vi "GetClassProperties.vi"(0 "reference in":refnum<class "ClassWriterGOOP300.lvclass">, 1 "LvClassItem":refnum<vi>, 2 "TreeControl":refnum<vi>, 5 "error in (no error)":errorcluster) -> (14 "reference out":refnum<class "ClassWriterGOOP300.lvclass">, 19 "error out":errorcluster)   [LabVIEW 2014, in "ClassWriterGOOP300.lvclass"]
uses:
  <resource>/Framework/Providers/Open_GDS/ClassProviders/Provider_EndevoGOOP300/ClassWriterGOOP300_class/ClassWriterGOOP300.lvclass
panel:
  out "ClassClasses":string[](array[string])
  out "ObjectClasses":string[](array[string])
  out "ClassAttributes":string[][](array[string])
  out "ObjectAttributes":string[][](array[string])
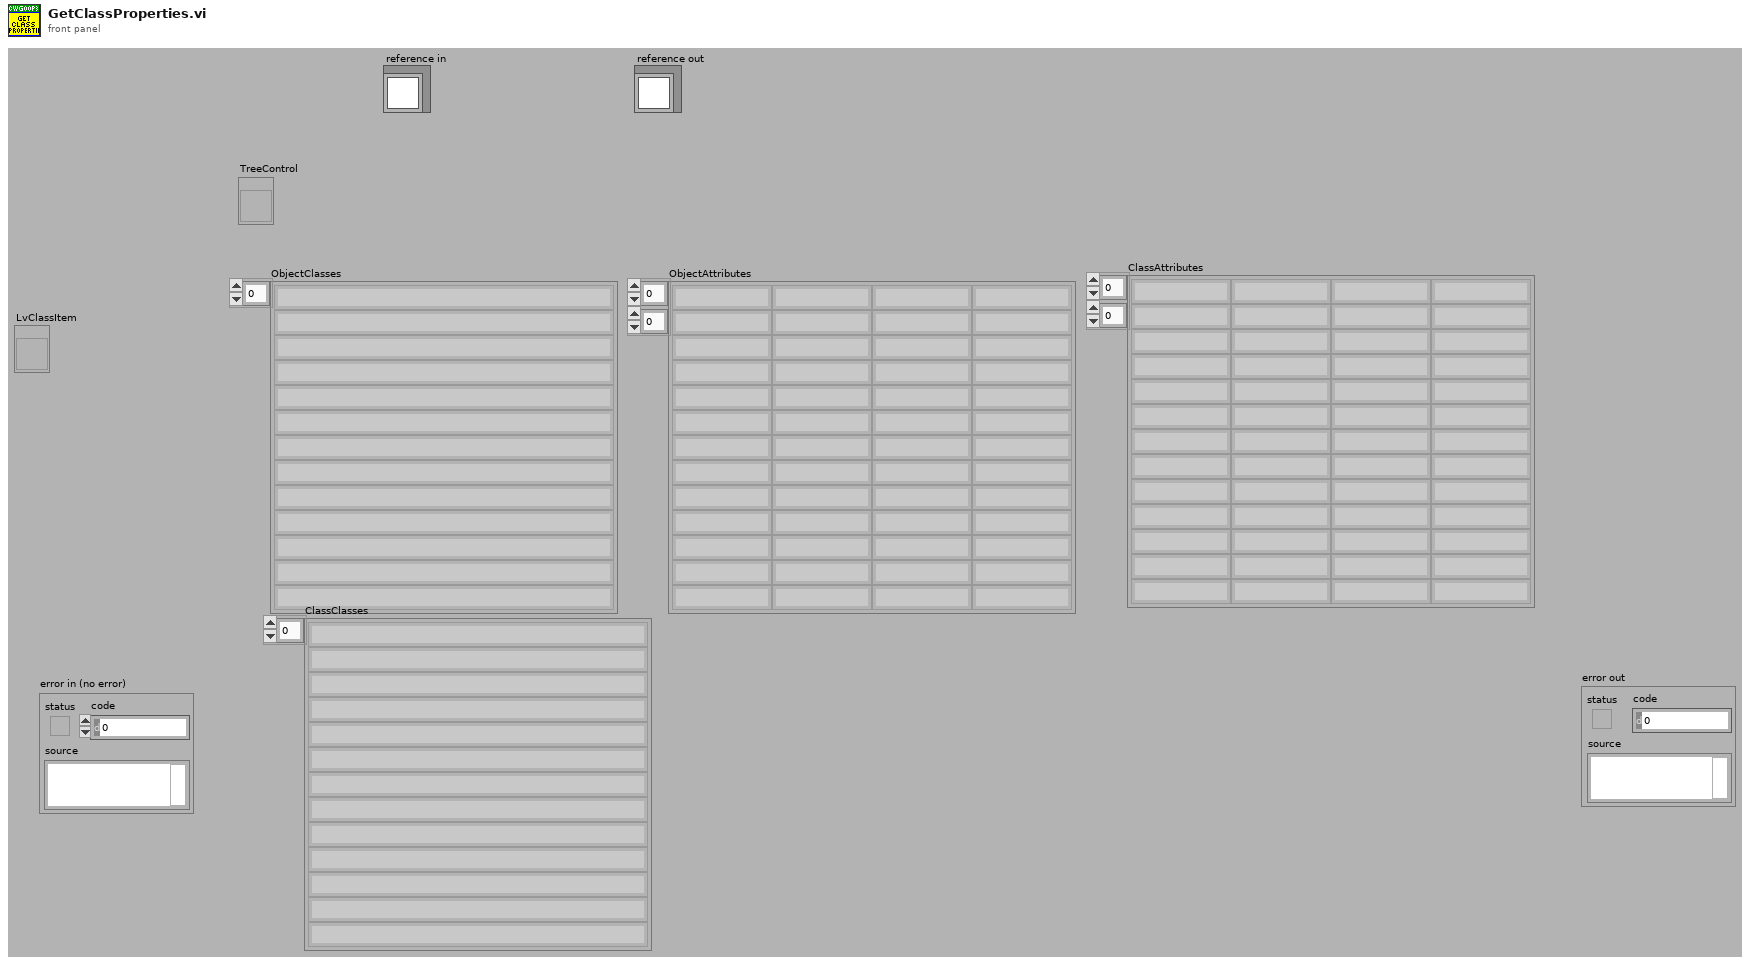
[diagram p1: front panel]
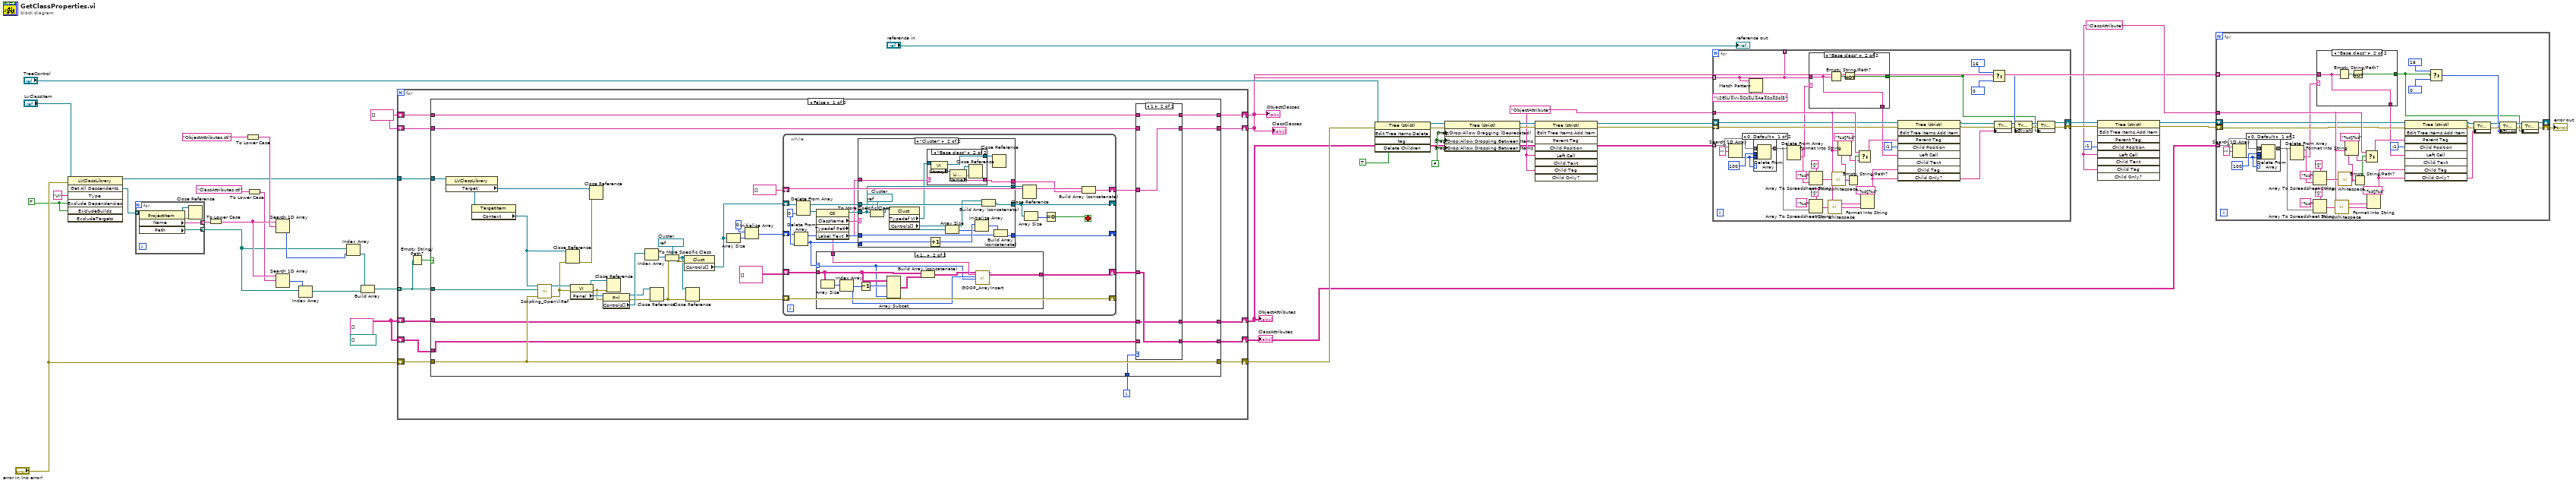
[diagram p0: block diagram]
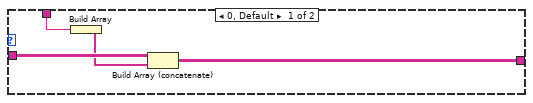
[diagram p7: hidden frame]
diagram:
  w2 = TRUE ("ExcludeDependencies")
  w10 = "ClassAttribute" ("Left Cell String(Main name)")
  w19 = FALSE ("Drag/Drop:Allow Dragging (Deprecated)")
  w13 = "ObjectAttribute" ("Left Cell String(Main name)")
  w25 = string[] []
  (unwired) path[] []
  w42 = string[][] []
  n1 = invoke class="LVClassLibrary" method="Get All Descendents"(reference="LvClassItem", error in="error in (no error)", "Type"="VI", "Exclude Dependencies"=w2, "ExcludeBuilds"=w2) -> (reference out=w1:refnum<vi>, "All Descendents"=w40:refnum<vi>[])  [unwired: 2 in, 5 out]
  n2 = for {
    tunnel: w40 -> [w48] mode=indexing
    tunnel: [w47] -> w39 mode=indexing
    tunnel: [w46] -> w33 mode=indexing
    n3 = property class="ProjectItem"(reference=w48) -> (reference out=w45:refnum<vi>, error out=w44:errorcluster, "Name"=w47:string, "Path"=w46:path)  [unwired: 1 in]
    n4 = Close Reference(reference=w45, error in (no error)=w44) -> ()  [unwired: 1 out]
  }
  n5 = To Lower Case(string=w39) -> (all lower case string=w37:string[])
  n6 = To Lower Case(string="ObjectAttributes.ctl") -> (all lower case string=w38:string)
  n7 = To Lower Case(string="ClassAttributes.ctl") -> (all lower case string=w36:string)
  n8 = Search 1D Array(1D array=w37, element=w38) -> (index of element=w35:i32)  [unwired: 1 in]
  n9 = Search 1D Array(1D array=w37, element=w36) -> (index of element=w34:i32)  [unwired: 1 in]
  n10 = Index Array(array=w33, index=w34) -> (element=w27:path)
  n11 = Index Array(array=w33, index=w35) -> (element=w28:path)
  n12 = Build Array(w28, w27) -> (w32:path[])
  n13 = for {
    shift-right: [w62] -> w7
    shift-left: "error in (no error)" -> [w61]
    shift-right: [w59] -> w6
    shift-left: w42 -> [w60]
    shift-right: [w57] -> w5
    shift-left: w42 -> [w58]
    tunnel: w32 -> [w56] mode=indexing
    shift-right: [w53] -> w4
    shift-left: w25 -> [w50]
    shift-right: [w52] -> w3
    shift-left: w25 -> [w51]
    tunnel: w1 -> [w49]
    i -> [w54]
    n14 = Empty String/Path?(string/path=w56) -> (empty?=w55:bool)
    n15 = case shown="False" w55 {
      tunnel: [w97 w171] -> w62
      tunnel: w61 -> [w97 w171]
      tunnel: w60 -> [w81 w172]
      tunnel: [w84 w172] -> w59
      tunnel: w58 -> [w83 w170]
      tunnel: [w82 w170] -> w57
      tunnel: w56 -> [w99 _]
      tunnel: w54 -> [w86 _]
      tunnel: [w72 w169] -> w53
      tunnel: [w70 w168] -> w52
      tunnel: w51 -> [w69 w168]
      tunnel: w50 -> [w68 w169]
      tunnel: w49 -> [w67 _]
      frame False {
        w90 = refnum<vi> refnum  # Cluster
        n16 = property class="LVClassLibrary"(reference=w67) -> ("Target"=w64:refnum<vi>)  [unwired: 1 in, 2 out]
        n17 = property class="TargetItem"(reference=w64) -> ("Context"=w66:refnum<vi>)  [unwired: 1 in, 2 out]
        n18 = call <resource>:"Scripting_OpenViRef.vi"("error in"=w97, "ViPath/ViName/Viref"=w99, "AppRef"=w66) -> ("error out"=w65:errorcluster, "vi reference"=w98:refnum<vi>)  [unwired: 6 in, 1 out]
        n19 = Close Reference(reference=w66, error in (no error)=w65) -> (error out=w63:errorcluster)
        n20 = property class="VI"(reference=w98, error in=w65) -> (reference out=w79:refnum<vi>, error out=w80:errorcluster, "Panel"=w96:refnum<vi>)
        n21 = Close Reference(reference=w64, error in (no error)=w63) -> ()  [unwired: 1 out]
        n22 = property class="Pnl"(reference=w96, error in=w80) -> (reference out=w74:refnum<vi>, error out=w76:errorcluster, "Controls[]"=w91:refnum<vi>[])
        n23 = Close Reference(reference=w79, error in (no error)=w80) -> ()  [unwired: 1 out]
        n24 = Index Array(array=w91) -> (element=w89:refnum<vi>)  [unwired: 1 in]
        n25 = Close Reference(reference=w74, error in (no error)=w76) -> (error out=w75:errorcluster)
        n26 = To More Specific Class(target class=w90, reference=w89, error in=w75) -> (specific class reference=w78:refnum<vi>, error out=w88:errorcluster)
        n27 = property class="Clust"(reference=w78, error in=w88) -> ("Controls[]"=w87:refnum<vi>[])  [unwired: 2 out]
        n28 = Close Reference(reference=w78, error in (no error)=w75) -> (error out=w77:errorcluster)
        n29 = Array Size(array=w87) -> (size(s)=w94:i32)
        n30 = Initialize Array(0 ("index"), w94) -> (w92:i32[])
        n31 = while {
          shift-right: [w126] -> _
          shift-left: w87 -> [w128]
          shift-right: [w113] -> _
          shift-left: w77 -> [w113]
          shift-right: [w121] -> w85
          shift-left: string[][] [] -> [w122]
          shift-right: [w115] -> _
          shift-left: w92 -> [w117]
          shift-right: [w110] -> w71
          shift-left: string[] [] -> [w111]
          stop <- w124 stop-if-true
          w118 = 0 ("index")
          n32 = Delete From Array(array=w117, index=w118) -> (deleted portion=w114:i32, array with subset deleted=w116:i32[])  [unwired: 1 in]
          n33 = Delete From Array(array=w128, index=w118) -> (deleted portion=w123:refnum<vi>, array with subset deleted=w127:refnum<vi>[])  [unwired: 1 in]
          n34 = property class="Ctl" props=["ClassName", "Typedef Path", "Label", "Text"](reference=w123) -> (reference out=w119:refnum<vi>, "ClassName"=w120:string, "Label.Text"=w108:string)  [unwired: 1 in, 2 out]
          n35 = case shown="1.." w114 {
            selector: w114 -> [_ w133]
            tunnel: w122 -> [w132 w137]
            tunnel: [w131 w140] -> w121
            tunnel: w108 -> [w130 w139]
            frame 0, Default {
              n36 = Build Array(w130) -> (w129:string[])
              n37 = Build Array (concatenate)(w132, w129) -> (w131:string[][])
            }
            frame 1.. {
              n38 = Array Size(array=w137) -> (size(s)=w141:i32[])
              n39 = Index Array(array=w141) -> (element=w135:i32)  [unwired: 1 in]
              n40 = Decrement(x=w135) -> (x-1=w134:i32)
              n41 = Array Subset(array=w137, index (row)=w134, length (col)=w133) -> (w136:string[][])  [unwired: 2 in]
              n42 = Build Array (concatenate)(w137, w136) -> (w138:string[][])
              n43 = call <resource>:"GOOP_ArrayInsert.vi"("ArrayIn"=w138, "Text"=w139, "Row"=w135, "Column"=w133) -> ("ArrayOut"=w140:string[][])  [unwired: 15 in]
            }
          }
          n44 = case shown="\"Cluster\"" w120 {
            tunnel: [w144 w158] -> w126
            tunnel: w127 -> [w144 w157]
            tunnel: w119 -> [w142 w149]
            tunnel: w116 -> [w143 w151]
            tunnel: [w143 w152] -> w115
            tunnel: w114 -> [_ w155]
            tunnel: [w142 w149] -> w112
            tunnel: [_ w147] -> w109
            tunnel: w108 -> [_ w145]
            frame Default {
            }
            frame "Cluster" {
              w160 = refnum<vi> refnum  # Cluster
              n45 = To More Specific Class(target class=w160, reference=w149) -> (specific class reference=w159:refnum<vi>)  [unwired: 1 in, 1 out]
              n46 = property class="Clust"(reference=w159) -> ("Typedef VI"=w148:refnum<vi>, "Controls[]"=w156:refnum<vi>[])  [unwired: 1 in, 2 out]
              n47 = case shown="\"Base class\"" w145 {
                tunnel: w148 -> [w161 w167]
                tunnel: [_ w165] -> w147
                tunnel: [w161 w162] -> w146
                frame "False", Default {
                }
                frame "Base class" {
                  n48 = property class="VI"(reference=w167) -> (reference out=w162:refnum<vi>, "Library"=w166:refnum<vi>)  [unwired: 1 in, 1 out]
                  n49 = property class="Library"(reference=w166) -> (reference out=w164:refnum<vi>, error out=w163:errorcluster, "Name"=w165:string)  [unwired: 1 in]
                  n50 = Close Reference(reference=w164, error in (no error)=w163) -> ()  [unwired: 1 out]
                }
              }
              n51 = Increment(x=w155) -> (x+1=w154:i32)
              n52 = Array Size(array=w156) -> (size(s)=w153:i32)
              n53 = Initialize Array(w154, w153) -> (w150:i32[])
              n54 = Build Array (concatenate)(w156, w157) -> (w158:refnum<vi>[])
              n55 = Close Reference(reference=w146) -> ()  [unwired: 1 in, 1 out]
              n56 = Build Array (concatenate)(w150, w151) -> (w152:i32[])
            }
          }
          n57 = Close Reference(reference=w112) -> ()  [unwired: 1 in, 1 out]
          n58 = Array Size(array=w126) -> (size(s)=w125:i32)
          n59 = Equal To 0?(x=w125) -> (x = 0?=w124:bool)
          n60 = Build Array (concatenate)(w111, w109) -> (w110:string[])
        }
        n61 = case shown="1" w86 {
          tunnel: [w103 w106] -> w84
          tunnel: w85 -> [w103 w107]
          tunnel: w83 -> [w102 _]
          tunnel: [w102 w107] -> w82
          tunnel: w81 -> [_ w106]
          tunnel: [w101 w105] -> w72
          tunnel: w71 -> [w101 w104]
          tunnel: [w100 w104] -> w70
          tunnel: w69 -> [w100 _]
          tunnel: w68 -> [_ w105]
          frame 0, Default {
          }
          frame 1 {
          }
        }
      }
      frame True {
      }
    }
  }
  "ObjectAttributes" <- w6
  "ClassAttributes" <- w5
  "ObjectClasses" <- w4
  "ClassClasses" <- w3
  n62 = invoke on="Invoke Node" class="Tree (strict)" method="Edit Tree Items.Delete"(reference="TreeControl", error in=w7, "Delete Children"=TRUE) -> (reference out=w23:refnum<vi>, error out=w22:errorcluster)  [unwired: 2 in, 3 out]
  n63 = property class="Tree (strict)"(reference=w23, error in=w22, "Drag/Drop:Allow Dragging (Deprecated)"=w19, "Drag/Drop:Allow Dropping Between Items"=w19, "Drag/Drop:Allow Dropping Between Items"=w19) -> (reference out=w21:refnum<vi>, error out=w20:errorcluster)
  n64 = invoke on="Invoke Node" class="Tree (strict)" method="Edit Tree Items.Add Item"(reference=w21, error in=w20, "Left Cell"=w13, "Child Tag"=w13) -> (reference out=w12:refnum<vi>, error out=w11:errorcluster)  [unwired: 5 in, 7 out]
  n65 = for {
    shift-right: [w175] -> w17
    shift-left: w11 -> [w192]
    shift-right: [w174] -> w18
    shift-left: w12 -> [w191]
    tunnel: w6 -> [w211] mode=indexing
    tunnel: w13 -> [w194]
    tunnel: w4 -> [w181] mode=indexing
    tunnel: [w181] -> _ mode=indexing
    n66 = Search 1D Array(1D array=w211, element="") -> (index of element=w200:i32)  [unwired: 1 in]
    n67 = Match Pattern(string=w181, regular expression="\\2E[Ll][Vv][Cc][Ll][Aa][Ss][Ss]$") -> ()  [unwired: 1 in, 4 out]
    n68 = case shown="0, Default" w200 {
      tunnel: w200 -> [w220 _]
      tunnel: w211 -> [w219 w221]
      tunnel: 100 ("length") -> [w218 _]
      tunnel: [w217 w221] -> w201
      frame 0, Default {
        n69 = Delete From Array(array=w219, length=w218, index=w220) -> (array with subset deleted=w217:string[])  [unwired: 1 out]
      }
      frame -1 {
      }
    }
    n70 = Delete From Array(array=w201) -> (deleted portion=w189:string, array with subset deleted=w209:string[])  [unwired: 2 in]
    n71 = case shown="\"Base class\"" w189 {
      selector: w189 -> [w213 _]
      tunnel: [w213 w214] -> w188
      tunnel: w181 -> [_ w214]
      tunnel: [_ w215] -> w173
      frame Default {
      }
      frame "Base class" {
        n72 = Empty String/Path?(string/path=w214) -> (empty?=w216:bool)
        n73 = Not(x=w216) -> (.not. x?=w215:bool)
      }
    }
    n74 = Array To Spreadsheet String(delimiter (Tab)="§", array=w209, 3:"%s" ("format string")) -> (spreadsheet string=w206:string)
    n75 = Array To Spreadsheet String(delimiter (Tab)="§", array=w201, 3:"%s" ("format string")) -> (spreadsheet string=w204:string)
    n76 = call <vilib>:"Trim Whitespace.vi"("string"=w204) -> ("trimmed string"=w195:string)  [unwired: 1 in]
    n77 = call <vilib>:"Trim Whitespace.vi"("string"=w206) -> ("trimmed string"=w198:string)  [unwired: 1 in]
    n78 = Format Into String(format string="%s§%s", w194, w198) -> (resulting string=w197:string)  [unwired: 2 in, 1 out]
    n79 = Empty String/Path?(string/path=w198) -> (empty?=w205:bool)
    n80 = Select(t=w194, s=w205, f=w197) -> (s? t:f=w193:string)
    n81 = Format Into String(format string="%s§%s", w194, w195) -> (resulting string=w182:string)  [unwired: 2 in, 1 out]
    n82 = invoke on="Invoke Node" class="Tree (strict)" method="Edit Tree Items.Add Item"(reference=w191, error in=w192, "Parent Tag"=w193, "Child Position"=-1, "Left Cell"=w188, "Child Tag"=w182) -> (reference out=w184:refnum<vi>, error out=w183:errorcluster)  [unwired: 3 in, 7 out]
    n83 = Select(t=16, s=w173, f=0) -> (s? t:f=w178:i32)
    n84 = property class="Tree (strict)"(reference=w184, error in=w183, "Active Item Tag"=w182) -> (reference out=w186:refnum<vi>, error out=w185:errorcluster)
    n85 = property class="Tree (strict)"(reference=w186, error in=w185, "Glyph"=w178) -> (reference out=w177:refnum<vi>, error out=w176:errorcluster)
    n86 = property class="Tree (strict)"(reference=w177, error in=w176, "Disabled?"=w173) -> (reference out=w174:refnum<vi>, error out=w175:errorcluster)
  }
  n87 = invoke on="Invoke Node" class="Tree (strict)" method="Edit Tree Items.Add Item"(reference=w18, error in=w17, "Child Position"=-1, "Left Cell"=w10, "Child Tag"=w10) -> (reference out=w9:refnum<vi>, error out=w8:errorcluster)  [unwired: 4 in, 7 out]
  n88 = for {
    shift-right: [w224] -> w16
    shift-left: w8 -> [w240]
    shift-right: [w223] -> _
    shift-left: w9 -> [w239]
    tunnel: w5 -> [w259] mode=indexing
    tunnel: w10 -> [w242]
    tunnel: w3 -> [w230] mode=indexing
    n89 = Search 1D Array(1D array=w259, element="") -> (index of element=w248:i32)  [unwired: 1 in]
    n90 = case shown="0, Default" w248 {
      tunnel: w248 -> [w268 _]
      tunnel: w259 -> [w267 w269]
      tunnel: 100 ("length") -> [w266 _]
      tunnel: [w265 w269] -> w249
      frame 0, Default {
        n91 = Delete From Array(array=w267, length=w266, index=w268) -> (array with subset deleted=w265:string[])  [unwired: 1 out]
      }
      frame -1 {
      }
    }
    n92 = Delete From Array(array=w249) -> (deleted portion=w237:string, array with subset deleted=w257:string[])  [unwired: 2 in]
    n93 = Array To Spreadsheet String(delimiter (Tab)="§", array=w257, 3:"%s" ("format string")) -> (spreadsheet string=w254:string)
    n94 = Array To Spreadsheet String(delimiter (Tab)="§", array=w249, 3:"%s" ("format string")) -> (spreadsheet string=w252:string)
    n95 = case shown="\"Base class\"" w237 {
      selector: w237 -> [w261 _]
      tunnel: [w261 w262] -> w236
      tunnel: w230 -> [_ w262]
      tunnel: [_ w263] -> w222
      frame Default {
      }
      frame "Base class" {
        n96 = Empty String/Path?(string/path=w262) -> (empty?=w264:bool)
        n97 = Not(x=w264) -> (.not. x?=w263:bool)
      }
    }
    n98 = call <vilib>:"Trim Whitespace.vi"("string"=w252) -> ("trimmed string"=w243:string)  [unwired: 1 in]
    n99 = call <vilib>:"Trim Whitespace.vi"("string"=w254) -> ("trimmed string"=w246:string)  [unwired: 1 in]
    n100 = Format Into String(format string="%s§%s", w242, w246) -> (resulting string=w245:string)  [unwired: 2 in, 1 out]
    n101 = Empty String/Path?(string/path=w246) -> (empty?=w253:bool)
    n102 = Select(t=w242, s=w253, f=w245) -> (s? t:f=w241:string)
    n103 = Format Into String(format string="%s§%s", w242, w243) -> (resulting string=w231:string)  [unwired: 2 in, 1 out]
    n104 = invoke on="Invoke Node" class="Tree (strict)" method="Edit Tree Items.Add Item"(reference=w239, error in=w240, "Parent Tag"=w241, "Child Position"=-1, "Left Cell"=w236, "Child Tag"=w231) -> (reference out=w233:refnum<vi>, error out=w232:errorcluster)  [unwired: 3 in, 7 out]
    n105 = Select(t=16, s=w222, f=0) -> (s? t:f=w228:i32)
    n106 = property class="Tree (strict)"(reference=w233, error in=w232, "Active Item Tag"=w231) -> (reference out=w235:refnum<vi>, error out=w234:errorcluster)
    n107 = property class="Tree (strict)"(reference=w235, error in=w234, "Glyph"=w228) -> (reference out=w226:refnum<vi>, error out=w225:errorcluster)
    n108 = property class="Tree (strict)"(reference=w226, error in=w225, "Disabled?"=w222) -> (reference out=w223:refnum<vi>, error out=w224:errorcluster)
  }
  "error out" <- w16
  "reference out" <- "reference in"
